vi "ActiView806-Lores.vi"() -> ()   [LabVIEW 2020] (continued)
          tunnel: [i32[] [1, 2, 3] ("Disabled Items []") i32[] [2, 3] ("Disabled Items []") i32[] [3] ("Disabled Items []") i32[] [] ("Disabled Items []") i32[] [1, 2, 3] ("Disabled Items []") i32[] [2, 3] ("Disabled Items []")] -> w1444
          tunnel: [u32 1 u32 3 u32 7 u32 15 u32 1 u32 3] -> w1438
          frame 0, Default {
          }
          frame 1 {
          }
          frame 2 {
          }
          frame 3 {
          }
          frame 14 {
          }
          frame 15 {
          }
        }
        n877 = local read "MonFreeAvg2"() -> (w1602:i32)
        n878 = local read "RefFreeAvg2"() -> (w1607:i32[])
        n879 = local read "MonFreeAvg1"() -> (w1597:i32)
        n880 = for {
          tunnel: w1584 -> [w2146]
          shift-right: [w2142] -> w1592
          shift-left: i32[] [] -> [w2144]
          tunnel: w1608 -> [w2140] mode=indexing
          n881 = Search 1D Array(1D array=w2146, element=w2140) -> (index of element=w2145:i32)  [unwired: 1 out]
          n882 = Greater Or Equal To 0?(x=w2145) -> (x >= 0?=w2143:bool)
          n883 = Build Array (concatenate)(w2144, w2140) -> (w2141:i32[])
          n884 = Select(t=w2141, s=w2143, f=w2144) -> (s? t:f=w2142:i32[])
        }
        n885 = for {
          tunnel: w1584 -> [w2139]
          shift-right: [w2135] -> w1586
          shift-left: i32[] [] -> [w2137]
          tunnel: w1607 -> [w2133] mode=indexing
          n886 = Search 1D Array(1D array=w2139, element=w2133) -> (index of element=w2138:i32)  [unwired: 1 out]
          n887 = Greater Or Equal To 0?(x=w2138) -> (x >= 0?=w2136:bool)
          n888 = Build Array (concatenate)(w2137, w2133) -> (w2134:i32[])
          n889 = Select(t=w2134, s=w2136, f=w2137) -> (s? t:f=w2135:i32[])
        }
        n890 = Search 1D Array(1D array=w1584, element=w1602) -> (index of element=w1604:i32)  [unwired: 1 out]
        n891 = Search 1D Array(1D array=w1584, element=w1597) -> (index of element=w1600:i32)  [unwired: 1 out]
        n892 = Greater Or Equal To 0?(x=w1604) -> (x >= 0?=w1603:bool)
        n893 = Greater Or Equal To 0?(x=w1600) -> (x >= 0?=w1599:bool)
        n894 = Select(t=w1438, s=w1439, f=u32 1) -> (s? t:f=w1440:u32)
        n895 = Select(t=w1602, s=w1603, f=0) -> (s? t:f=w1595:i32)
        n896 = Select(t=w1597, s=w1599, f=0) -> (s? t:f=w1596:i32)
        n897 = property on="Box" class="Ring (strict)"("Visible"=w1439, "Disabled Items []"=w1444) -> ()  [unwired: 2 in, 2 out]
        n898 = Bundle By Name(cluster=w1442, "Save Box"=w1440) -> (w1441:T7)
        n899 = Array Size(array=w1592) -> (size(s)=w1594:i32)
        n900 = Array Size(array=w1586) -> (size(s)=w1589:i32)
        n901 = Equal To 0?(x=w1594) -> (x = 0?=w1593:bool)
        n902 = Equal To 0?(x=w1589) -> (x = 0?=w1588:bool)
        n903 = Select(t=i32[] [0], s=w1593, f=w1592) -> (s? t:f=w1591:i32[])
        n904 = Select(t=i32[] [0], s=w1588, f=w1586) -> (s? t:f=w1585:i32[])
        n905 = case shown="True" w1625 {
          tunnel: w1647 -> [_ w2249]
          tunnel: w1579 -> [_ w2248]
          tunnel: w1578 -> [_ w2247]
          tunnel: w1613 -> [_ w2246]
          tunnel: w1639 -> [_ w2245]
          tunnel: w1577 -> [_ w2244]
          tunnel: w1643 -> [_ w2243]
          tunnel: w1636 -> [_ w2242]
          tunnel: w1596 -> [_ w2241]
          tunnel: w1591 -> [_ w2240]
          tunnel: w1595 -> [_ w2239]
          tunnel: w1585 -> [_ w2238]
          tunnel: w1574 -> [_ w2235]
          tunnel: w1573 -> [_ w2237]
          tunnel: w1439 -> [_ w2233]
          tunnel: w1474 -> [_ w2231]
          frame False {
          }
          frame True {
            w2236 = i8 7 items=["A1 - H32 (256)", "A1 - E32 (160)", "A1 - D32 (128)", "A1 - B32 (64)", "A1 - A32 (32)", "A1 - A16 (16)", "A1 -A8 (8)", "None (0) "] ("TCPsubset")
            n906 = local write "Channels"(w2249) -> ()
            n907 = local write "Offset"(w2245) -> ()
            n908 = local write "Reference"(w2243) -> ()
            n909 = property on="Channels" class="Ring (strict)"("Disabled Items []"=w2248) -> ()  [unwired: 2 in, 2 out]
            n910 = property on="Reference" class="Ring (strict)"("Disabled Items []"=w2247) -> ()  [unwired: 2 in, 2 out]
            n911 = property on="Offset" class="Ring (strict)"("Disabled Items []"=w2244) -> ()  [unwired: 2 in, 2 out]
            n912 = property on="TCPsubset" class="Ring (strict)"("Disabled Items []"=w2237) -> ()  [unwired: 2 in, 2 out]
            n913 = local write "MonFree"(w2246) -> ()
            n914 = Select(t=w2236, s=w2233, f=w2235) -> (s? t:f=w2234:i8)
            n915 = local write "RefFree"(w2242) -> ()
            n916 = local write "TCPsubset"(w2234) -> ()
            n917 = local write "MonFreeAvg1"(w2241) -> ()
            n918 = local read "AddTP"() -> (w2229:bool)
            n919 = local write "RefFreeAvg1"(w2240) -> ()
            n920 = local write "Charts/Graphs"(T2."Monopolar Display" ("Charts/Graphs")) -> ()
            n921 = local write "MonFreeAvg2"(w2239) -> ()
            n922 = And(x=w2229, y=w2231) -> (x .and. y?=w2230:bool)
            n923 = local write "AddTP"(w2230) -> ()
            n924 = local write "RefFreeAvg2"(w2238) -> ()
          }
        }
        n925 = local read "TCPaddTP"() -> (w1534:bool)
        n926 = local read "TCPaddAnas"() -> (w1530:bool)
        n927 = local read "TCPaddTrig"() -> (w1526:bool)
        n928 = local read "TCPaddSens"() -> (w1532:bool)
        n929 = local read "TCPaddJazz"() -> (w1473:bool)
        n930 = local read "Averaging"() -> (w1528:bool)
        n931 = Not(x=w1439) -> (.not. x?=w1472:bool)
        n932 = And(x=w1472, y=w1528) -> (x .and. y?=w1527:bool)
        n933 = Compound Arithmetic op=AND(w1534, w1474, w1472) -> (w1533:bool)
        n934 = Compound Arithmetic op=AND(w1532, w1474, w1472) -> (w1531:bool)
        n935 = Compound Arithmetic op=AND(w1530, w1496, w1472) -> (w1529:bool)
        n936 = And(x=w1526, y=w1472) -> (x .and. y?=w1525:bool)
        n937 = Compound Arithmetic op=AND(w1473, w1470, w1472) -> (w1471:bool)
        n938 = local write "Averaging"(w1527) -> ()
        n939 = local write "TCPaddTP"(w1533) -> ()
        n940 = local write "TCPaddAnas"(w1529) -> ()
        n941 = local write "TCPaddTrig"(w1525) -> ()
        n942 = local write "TCPaddSens"(w1531) -> ()
        n943 = local write "TCPaddJazz"(w1471) -> ()
        n944 = property on="Charts/Graphs" class="TabCtl (strict)"() -> ("Pages"=w1557:refnum<vi>[])  [unwired: 2 in, 2 out]
        n945 = Index Array(array=w1557, index #1=1 ("index")) -> (element #1=w1550:refnum<vi>, element #3=w1536:refnum<vi>, element #4=w1549:refnum<vi>, element #5=w1491:refnum<vi>, element #6=w1492:refnum<vi>, element #7=w1535:refnum<vi>)  [unwired: 6 in, 1 out]
        n946 = Array Size(array=w1569) -> (size(s)=w1635:i32)
        n947 = Unbundle By Name(w1633) -> ("All Labels"=w1486:string[])
        n948 = Not Equal To 0?(x=w1635) -> (x != 0?=w1634:bool)
        n949 = Unbundle By Name(w1441) -> ("Mon Channels"=w1658:i32, "Bip Channels"=w1657:i32, "Aux Channels"=w1567:i32, "Jazz Channels"=w1485:i32, "Ana Channels"=w1490:i32)
        n950 = And(x=w1634, y=w1474) -> (x .and. y?=w1541:bool)
        n951 = Array Size(array=w1542) -> (size(s)=w1559:i32)
        n952 = Array Size(array=w1480) -> (size(s)=w1481:i32)
        n953 = Array Size(array=w1543) -> (size(s)=w1561:i32)
        n954 = property on="Ring Buffer" class="Knob (strict)"("Scale.Uniform Marker Spacing?"=FALSE) -> ()  [unwired: 2 in, 2 out]
        n955 = Not Equal To 0?(x=w1481) -> (x != 0?=w1478:bool)
        n956 = Not Equal To 0?(x=w1559) -> (x != 0?=w1558:bool)
        n957 = Not Equal To 0?(x=w1561) -> (x != 0?=w1560:bool)
        n958 = Array Size(array=w1486) -> (size(s)=w1632:i32)
        n959 = Select(t=T5."Enabled" ("Disabled"), s=w1541, f=T5."Disabled and Grayed Out" ("Disabled")) -> (s? t:f=w1568:T5)
        n960 = And(x=w1560, y=w1496) -> (x .and. y?=w1545:bool)
        n961 = And(x=w1478, y=w1470) -> (x .and. y?=w1479:bool)
        n962 = And(x=w1558, y=w1474) -> (x .and. y?=w1551:bool)
        n963 = Select(t=T4."Page Enabled" ("Page Enabled State"), s=w1541, f=T4."Page Disabled & Grayed" ("Page Enabled State")) -> (s? t:f=w1555:T4)
        n964 = Select(t=T4."Page Enabled" ("Page Enabled State"), s=w1479, f=T4."Page Disabled & Grayed" ("Page Enabled State")) -> (s? t:f=w1497:T4)
        n965 = Decrement(x=w1632) -> (x-1=w1631:i32)
        n966 = Select(t=T4."Page Enabled" ("Page Enabled State"), s=w1545, f=T4."Page Disabled & Grayed" ("Page Enabled State")) -> (s? t:f=w1546:T4)
        n967 = Select(t=T4."Page Enabled" ("Page Enabled State"), s=w1551, f=T4."Page Disabled & Grayed" ("Page Enabled State")) -> (s? t:f=w1548:T4)
        n968 = Select(t=T4."Page Enabled" ("Page Enabled State"), s=w1472, f=T4."Page Disabled & Grayed" ("Page Enabled State")) -> (s? t:f=w1537:T4)
        n969 = property on="TP Offset Graph 1" class="WFGraph (strict)"("Disabled"=w1568) -> ()  [unwired: 2 in, 2 out]
        n970 = property on="TP Offset Graph 2" class="WFGraph (strict)"("Disabled"=w1568) -> ()  [unwired: 2 in, 2 out]
        n971 = Index Array(array=w1486, index=w1631) -> (element=w1489:string)
        n972 = property class="Page"(reference=w1550, "Page Enabled State"=w1555) -> ()  [unwired: 1 in, 2 out]
        n973 = property class="Page"(reference=w1549, "Page Enabled State"=w1548) -> ()  [unwired: 1 in, 2 out]
        n974 = property class="Page"(reference=w1491, "Page Enabled State"=w1497) -> ()  [unwired: 1 in, 2 out]
        n975 = property class="Page"(reference=w1492, "Page Enabled State"=w1546) -> ()  [unwired: 1 in, 2 out]
        n976 = property class="Page"(reference=w1536, "Page Enabled State"=w1537) -> ()  [unwired: 1 in, 2 out]
        n977 = property class="Page"(reference=w1535, "Page Enabled State"=w1537) -> ()  [unwired: 1 in, 2 out]
        n978 = Array Subset(array=w1486, length=w1658) -> (w1663:string[])  [unwired: 1 in]
        n979 = Array Subset(array=w1486, index=256, length=w1657) -> (w1662:string[])
        n980 = Array Subset(array=w1486, index=264, length=w1567) -> (w1659:string[])
        n981 = Array Subset(array=w1486, index=272, length=w1485) -> (w1487:string[])
        n982 = Array Subset(array=w1486, index=281, length=w1490) -> (w1488:string[])
        n983 = Build Array (concatenate)(w1663, w1662, w1659, w1487, w1488, w1489) -> (w1630:string[])
        n984 = for {
          N: w1464 -> [_]
          tunnel: w1630 -> [w2251] mode=indexing
          tunnel: [w2250] -> w1672 mode=indexing
          n985 = String Subset(string=w2251, length (rest)=4 ("length (rest)")) -> (substring=w2250:string)  [unwired: 1 out]
        }
        n986 = for {
          tunnel: w1630 -> [w2219] mode=indexing
          tunnel: [w2218] -> w1628 mode=indexing
          n987 = Format Into String(format string="%-16.16s", w2219) -> (resulting string=w2218:string)  [unwired: 2 in, 1 out]
        }
        n988 = property on="MonFree" class="LstBox (strict)"("Item Names"=w1672) -> ()  [unwired: 2 in, 2 out]
        n989 = property on="RefFree" class="LstBox (strict)"("Item Names"=w1672) -> ()  [unwired: 2 in, 2 out]
        n990 = Bundle By Name(cluster=w1633, "Spec Labels"=w1628) -> (w1629:T8)
        n991 = Select(t=T5."Enabled" ("Disabled"), s=w1474, f=T5."Disabled and Grayed Out" ("Disabled")) -> (s? t:f=w1671:T5)
        n992 = property on="RefFreeAvg1" class="LstBox (strict)"("Item Names"=w1672) -> ()  [unwired: 2 in, 2 out]
        n993 = property on="MonFreeAvg1" class="LstBox (strict)"("Item Names"=w1672) -> ()  [unwired: 2 in, 2 out]
        n994 = property on="Battery\nCapacitance" class="Slide (strict)"("Disabled"=w1671) -> ()  [unwired: 2 in, 2 out]
        n995 = property on="RefFreeAvg2" class="LstBox (strict)"("Item Names"=w1672) -> ()  [unwired: 2 in, 2 out]
        n996 = property on="MonFreeAvg2" class="LstBox (strict)"("Item Names"=w1672) -> ()  [unwired: 2 in, 2 out]
      }
      frame 2 {
        w2260 = T5."Disabled and Grayed Out" ("Disabled")
        w2294 = 5  # Go to State 5:    stop running
        w2266 = FALSE
        w2261 = FALSE
        w2278 = 0 ("Dimension Size")
        w2307 = FALSE  # Stop Running
        w2310 = 4  # Go to State 4    Displaying
        w2311 = 3  # Go to State 3     Saving
        # "Screen Duration"
        # "Sample Rate"
        # "Busy Saving"
        n997 = flat-sequence {
          tunnel: w2273 -> [w2318]
          tunnel: w2271 -> [w2317]
          tunnel: w2272 -> [w2316]
          tunnel: w2271 -> [w2323]
          tunnel: w2271 -> [w2328]
          frame #0 {
            w2314 = 0 ("Dimension Size")
            # "Cear the Charts"
            n998 = Initialize Array(w2314, w2314, w2314) -> (w2313:i32[][])
            n999 = To Double Precision Float(number=w2313) -> (double precision float=w2312:dbl[][])
            n1000 = property on="Trigger Chart" class="WFChart (strict)"("History Data"=w2313) -> ()  [unwired: 2 in, 2 out]
            n1001 = property on="Mon Chart" class="WFChart (strict)"("History Data"=w2312) -> ()  [unwired: 2 in, 2 out]
            n1002 = property on="Bip Chart" class="WFChart (strict)"("History Data"=w2312) -> ()  [unwired: 2 in, 2 out]
            n1003 = property on="Aux Chart" class="WFChart (strict)"("History Data"=w2312) -> ()  [unwired: 2 in, 2 out]
            n1004 = property on="Jazz Chart" class="WFChart (strict)"("History Data"=w2312) -> ()  [unwired: 2 in, 2 out]
            n1005 = property on="Ana Chart" class="WFChart (strict)"("History Data"=w2312) -> ()  [unwired: 2 in, 2 out]
          }
          frame #1 {
            # "Scale the Charts"
            # "Set \"Chart History Lenght\" at:\n(x-scale lenghts in s) * (sample rate) + 1"
            # "Sample Rate on screen"
            n1006 = Multiply(x=w2316, y=w2317) -> (x*y=w2321:i32)
            n1007 = Quotient & Remainder(x=w2318, y=w2321) -> (floor(x/y)=w2320:i32)  [unwired: 1 out]
            n1008 = To Double Precision Float(number=w2320) -> (double precision float=w2319:dbl)
            n1009 = Reciprocal(x=w2319) -> (1/x=w2315:dbl)
            n1010 = property on="Mon Chart" class="WFChart (strict)"("X Scale.Offset and Multiplier:Multiplier"=w2315) -> ()  [unwired: 2 in, 2 out]
            n1011 = property on="Trigger Chart" class="WFChart (strict)"("X Scale.Offset and Multiplier:Multiplier"=w2315) -> ()  [unwired: 2 in, 2 out]
            n1012 = property on="Bip Chart" class="WFChart (strict)"("X Scale.Offset and Multiplier:Multiplier"=w2315) -> ()  [unwired: 2 in, 2 out]
            n1013 = property on="Aux Chart" class="WFChart (strict)"("X Scale.Offset and Multiplier:Multiplier"=w2315) -> ()  [unwired: 2 in, 2 out]
            n1014 = property on="Jazz Chart" class="WFChart (strict)"("X Scale.Offset and Multiplier:Multiplier"=w2315) -> ()  [unwired: 2 in, 2 out]
            n1015 = property on="Ana Chart" class="WFChart (strict)"("X Scale.Offset and Multiplier:Multiplier"=w2315) -> ()  [unwired: 2 in, 2 out]
          }
          frame #2 {
            n1016 = To Double Precision Float(number=w2323) -> (double precision float=w2322:dbl)
            n1017 = property on="Mon Chart" class="WFChart (strict)"("X Scale.Range:Maximum"=w2322) -> ()  [unwired: 2 in, 2 out]
            n1018 = property on="Trigger Chart" class="WFChart (strict)"("X Scale.Range:Maximum"=w2322) -> ()  [unwired: 2 in, 2 out]
            n1019 = property on="Bip Chart" class="WFChart (strict)"("X Scale.Range:Maximum"=w2322) -> ()  [unwired: 2 in, 2 out]
            n1020 = property on="Aux Chart" class="WFChart (strict)"("X Scale.Range:Maximum"=w2322) -> ()  [unwired: 2 in, 2 out]
            n1021 = property on="Jazz Chart" class="WFChart (strict)"("X Scale.Range:Maximum"=w2322) -> ()  [unwired: 2 in, 2 out]
            n1022 = property on="Ana Chart" class="WFChart (strict)"("X Scale.Range:Maximum"=w2322) -> ()  [unwired: 2 in, 2 out]
          }
          frame #3 {
            n1023 = Greater Or Equal?(x=1, y=w2328) -> (x >= y?=w2327:bool)
            n1024 = Select(t=u8 1, s=w2327, f=u8 0) -> (s? t:f=w2324:u8)
            n1025 = property on="Mon Chart" class="WFChart (strict)"("X Scale.Format & Precision:Precision"=w2324) -> ()  [unwired: 2 in, 2 out]
            n1026 = property on="Bip Chart" class="WFChart (strict)"("X Scale.Format & Precision:Precision"=w2324) -> ()  [unwired: 2 in, 2 out]
            n1027 = property on="Aux Chart" class="WFChart (strict)"("X Scale.Format & Precision:Precision"=w2324) -> ()  [unwired: 2 in, 2 out]
            n1028 = property on="Jazz Chart" class="WFChart (strict)"("X Scale.Format & Precision:Precision"=w2324) -> ()  [unwired: 2 in, 2 out]
            n1029 = property on="Ana Chart" class="WFChart (strict)"("X Scale.Format & Precision:Precision"=w2324) -> ()  [unwired: 2 in, 2 out]
          }
        }
        n1030 = Unbundle By Name(w2267) -> ("ADC Rate"=w2273:i32, "Screen Ratio"=w2272:i32)
        n1031 = for {
          N: 9 -> [_]
          tunnel: w2300 -> [w2353]
          tunnel: [w2349] -> w2301 mode=indexing
          i -> [w2354]
          n1032 = Multiply(x=w2353, y=w2354) -> (x*y=w2352:i32)
          n1033 = To Double Precision Float(number=w2352) -> (double precision float=w2351:dbl)
          n1034 = Bundle(w2351, u32 0) -> (w2349:cluster{dbl, u32})  [unwired: 1 out]
        }
        n1035 = property on="Ring Buffer" class="Knob (strict)"("Scale.Marker Values[]"=w2301) -> ()  [unwired: 2 in, 2 out]
        n1036 = property on="ScreenLength" class="Ring (strict)"("Disabled"=w2260) -> ()  [unwired: 2 in, 2 out]
        n1037 = property on="Decimation" class="Ring (strict)"("Disabled"=w2260) -> ()  [unwired: 2 in, 2 out]
        n1038 = property on="Buffer" class="Ring (strict)"("Disabled"=w2260) -> ()  [unwired: 2 in, 2 out]
        n1039 = property on="Load Configuration File" class="Bool"("Disabled"=w2260) -> ()  [unwired: 2 in, 2 out]
        n1040 = property on="Save Configuration File" class="Bool"("Disabled"=w2260) -> ()  [unwired: 2 in, 2 out]
        n1041 = property on="Edit" class="Bool"("Disabled"=w2260) -> ()  [unwired: 2 in, 2 out]
        n1042 = property on="LocalPort" class="DigNum (strict)"("Disabled"=w2260) -> ()  [unwired: 2 in, 2 out]
        n1043 = property on="TCPsubset" class="Ring (strict)"("Disabled"=w2260) -> ()  [unwired: 2 in, 2 out]
        n1044 = property on="TCPaddTP" class="Bool (strict)"("Disabled"=w2260) -> ()  [unwired: 2 in, 2 out]
        n1045 = property on="TCPaddSens" class="Bool (strict)"("Disabled"=w2260) -> ()  [unwired: 2 in, 2 out]
        n1046 = property on="TCPaddAnas" class="Bool (strict)"("Disabled"=w2260) -> ()  [unwired: 2 in, 2 out]
        n1047 = property on="TCPaddJazz" class="Bool (strict)"("Disabled"=w2260) -> ()  [unwired: 2 in, 2 out]
        n1048 = property on="TCPaddTrig" class="Bool (strict)"("Disabled"=w2260) -> ()  [unwired: 2 in, 2 out]
        n1049 = property on="JazzOn" class="Bool (strict)"("Disabled"=w2260) -> ()  [unwired: 2 in, 2 out]
        n1050 = global write "TCPidentification.glb" "TCP cluster"(T9 {"connection ID"=refnum, "remote address"="", "remote port"=0} ("TCP cluster")) -> ()
        n1051 = local write "Save Subset"("" ("Local Patient Identification")) -> ()
        n1052 = local write "with  8 EX"(w2266) -> ()
        n1053 = local write "with Sens"(w2266) -> ()
        n1054 = local write "with AIB"(w2266) -> ()
        n1055 = local write "RejAbs"(w2266) -> ()
        n1056 = local write "RejDif"(w2266) -> ()
        n1057 = local write "Box1"(w2266) -> ()
        n1058 = local write "Box2"(w2266) -> ()
        n1059 = local write "Box3"(w2266) -> ()
        n1060 = local write "Box4"(w2266) -> ()
        n1061 = Greater Than 0?(x=w2277) -> (x > 0?=w2276:bool)
        n1062 = Unbundle By Name(w2267) -> ("Mon Channels"=w2292:i32, "Bip Channels"=w2291:i32)
        n1063 = property on="MonFree" class="LstBox (strict)"() -> ("Item Names"=w2282:string[])  [unwired: 2 in, 2 out]
        n1064 = To Double Precision Float(number=w2278) -> (double precision float=w2281:dbl)
        n1065 = local write "Total Saved sec"(w2278) -> ()
        n1066 = case shown="True" w2276 {
          tunnel: w2277 -> [_ w2342]
          frame False {
          }
          frame True {
            n1067 = Divide(x=w2342, y=2.0) -> (x/y=w2344:dbl)
            n1068 = Decrement(x=w2344) -> (x-1=w2332:dbl)
            n1069 = property on="BipLPfreq" class="DigNum (strict)"("Data Range:Maximum"=w2332) -> ()  [unwired: 2 in, 2 out]
            n1070 = property on="AvgLPfreq" class="DigNum (strict)"("Data Range:Maximum"=w2332) -> ()  [unwired: 2 in, 2 out]
            n1071 = property on="MonLPfreq" class="DigNum (strict)"("Data Range:Maximum"=w2332) -> ()  [unwired: 2 in, 2 out]
            n1072 = property on="AnaHPfreq" class="DigNum (strict)"("Data Range:Maximum"=w2332) -> ()  [unwired: 2 in, 2 out]
            n1073 = local read "MonLPfreq"() -> (w2341:dbl)
            n1074 = local read "AvgLPfreq"() -> (w2335:dbl)
            n1075 = local read "AnaLPfreq"() -> (w2331:dbl)
            n1076 = local read "BipLPfreq"() -> (w2338:dbl)
            n1077 = Less Or Equal?(x=w2338, y=w2332) -> (x <= y?=w2339:bool)
            n1078 = Less Or Equal?(x=w2341, y=w2332) -> (x <= y?=w2345:bool)
            n1079 = Less Or Equal?(x=w2335, y=w2332) -> (x <= y?=w2336:bool)
            n1080 = Less Or Equal?(x=w2331, y=w2332) -> (x <= y?=w2333:bool)
            n1081 = Select(t=w2338, s=w2339, f=w2332) -> (s? t:f=w2337:dbl)
            n1082 = Select(t=w2341, s=w2345, f=w2332) -> (s? t:f=w2340:dbl)
            n1083 = Select(t=w2335, s=w2336, f=w2332) -> (s? t:f=w2334:dbl)
            n1084 = Select(t=w2331, s=w2333, f=w2332) -> (s? t:f=w2330:dbl)
            n1085 = local write "MonLPfreq"(w2340) -> ()
            n1086 = local write "BipLPfreq"(w2337) -> ()
            n1087 = local write "AnaLPfreq"(w2330) -> ()
            n1088 = local write "AvgLPfreq"(w2334) -> ()
          }
        }
        n1089 = global write "LoBatWarning.glb" "LoBatWarning"(w2261) -> ()
        n1090 = global write "JazzLoBatWarning.glb" "JazzLoBatWarning"(w2261) -> ()
        n1091 = Format Into String(format string="%-4.4s", "" ("input 1")) -> (resulting string=w2284:string)  [unwired: 2 in, 1 out]
        n1092 = global write "StopThreads.glb" "StopThreads"(w2261) -> ()
        n1093 = property class="VI"("Front Panel Window:Closeable"=FALSE) -> ()  [unwired: 2 in, 2 out]
        n1094 = local write "Current File MB"(w2281) -> ()
        n1095 = Build Array (concatenate)(w2282, w2284) -> (w2288:string[])
        n1096 = Add(x=w2292, y=w2291) -> (x+y=w2290:i32)
        n1097 = Match First String(2:w2288, 3:w2284) -> (0:w2289:i32)  [unwired: 1 out]
        n1098 = Not Equal?(x=w2289, y=w2290) -> (x != y?=w2283:bool)
        n1099 = Build Array(FALSE ("element"), w2283, FALSE ("element")) -> (w2303:bool[])
        n1100 = case shown="True" w2262 {
          selector: w2262 -> [_ w2346]
          frame False {
          }
          frame True {
            n1101 = flat-sequence {
              tunnel: w2346 -> [w2347]
              frame #0 {
                n1102 = local write "Start Saving"(w2347) -> ()
              }
              frame #1 {
                n1103 = property on="Start Saving" class="Bool (strict)"("Boolean Text.Text"="Initializing") -> ()  [unwired: 2 in, 2 out]
              }
            }
          }
        }
        n1104 = Boolean Array To Number(Boolean array=w2303) -> (number=w2298:u32)
        n1105 = call "Act_ConfigError.vi"("Error Code In"=w2298, "error in (no error)"=w2297) -> ("error out"=w2264:errorcluster)  [unwired: 2 out]
        n1106 = Unbundle By Name(w2264) -> ("status"=w2296:bool)
        n1107 = Select(t=w2311, s=w2262, f=w2310) -> (s? t:f=w2295:i32)
        n1108 = Select(t=w2294, s=w2296, f=w2295) -> (s? t:f=w2293:i32)
      }
      frame 3 {
        w2411 = 43 items=["No Error", "Manager Argument Error", "Memory Full", "Out of Zone", "End of File", "File Already Open", "Generic File IO Error", "File Not Found", "File Permission Error", "Disk Full", "Duplicate Path", "Too Many Files Open", "Not Enabled", "Resource File Not Found", "Cannot Add Resource", "Resource Not Found", "Image Not Found", "Image Memory Error", "Pen Does Not Exist", "Config Bad Type", "Config Token Not Found", "Config Parse Error", "Config Memory Error", "Bad External Code Format", "Bad External Code Offset", "External Code Not Present", "Null Window", "Destroy Window Mixup", "Null Menu", "Print Aborted", "Bad Print Record", "Print Driver Error", "Windows Error During Print", "Memory Error During Print", "Print Dialog Error", "Generic Print Error", "Invalid Device Refnum", "Device Not Found", "Device Parameter Error", "Device Unit Error", "Can't Open Device", "Device Call Aborted", "Generic Error", "Cancelled By User"]
        w2426 = 43 items=["No Error", "Manager Argument Error", "Memory Full", "Out of Zone", "End of File", "File Already Open", "Generic File IO Error", "File Not Found", "File Permission Error", "Disk Full", "Duplicate Path", "Too Many Files Open", "Not Enabled", "Resource File Not Found", "Cannot Add Resource", "Resource Not Found", "Image Not Found", "Image Memory Error", "Pen Does Not Exist", "Config Bad Type", "Config Token Not Found", "Config Parse Error", "Config Memory Error", "Bad External Code Format", "Bad External Code Offset", "External Code Not Present", "Null Window", "Destroy Window Mixup", "Null Menu", "Print Aborted", "Bad Print Record", "Print Driver Error", "Windows Error During Print", "Memory Error During Print", "Print Dialog Error", "Generic Print Error", "Invalid Device Refnum", "Device Not Found", "Device Parameter Error", "Device Unit Error", "Can't Open Device", "Device Call Aborted", "Generic Error", "Cancelled By User"]
        w2441 = FALSE  # Stop Running
        # "Jazz Chan Selection"
        # "Ana Chan Selection"
        # "Aux Chan Selection"
        # "Mon Chan Selection"
        # "path does exist"
        # "Current File in Byte"
        # "Header Lenght in Byte"
        n1109 = Unbundle By Name(w2414) -> ("Save Path"=w2362:path, "Mark2"=w2374:bool, "GSR16Hz"=w2373:bool, "Jazz Channels"=w2372:i32, "Speed Mode"=w2364:i8, "ADC Rate"=w2418:i32, "Decimate Ratio"=w2419:i32, "Mon Channels"=w2400:i32, "Bip Channels"=w2399:i32, "Save Subset"=w2398:i8, "Add Touchproofs"=w2397:bool, "Add Sensors"=w2393:bool, "Add Jazz"=w2379:bool, "Add Anas"=w2380:bool, "Save Box"=w2381:u32)
        n1110 = Not Equal To 0?(x=w2372) -> (x != 0?=w2367:bool)
        n1111 = call "AVTCP-Local ID FGV.vi"() -> ("Value out"=w2357:cluster{"subj":string, "rec":string}, "not empty"=w2358:bool)  [unwired: 6 in]
        n1112 = Bundle("Save Subset"=w2398, "Add Touchproofs"=w2397, "Add Sensors"=w2393, "Add Jazz"=w2379, "Add Anas"=w2380, "Save Box"=w2381) -> (w2424:T20)  [unwired: 1 out]
        n1113 = case shown="False" w2358 {
          tunnel: [w2453 w2455] -> w2437
          tunnel: w2424 -> [w2452 w2456]
          tunnel: [w2451 w2456] -> w2413
          tunnel: [w2450 "Default" ("Save Subset")] -> w2406
          tunnel: w2374 -> [w2449 _]
          tunnel: [w2448 _] -> w2368
          tunnel: w2367 -> [w2447 _]
          tunnel: w2364 -> [w2446 _]
          tunnel: w2357 -> [_ w2455]
          frame False {
            n1114 = call "BDFlocal-Daisy.vi"("Mark2"=w2449, "JazzOn"=w2447, "Speedmode"=w2446, "Default Save Cluster"=w2452) -> ("Save Subset"=w2450:string, "Local ID"=w2453:T21, "Save Cluster"=w2451:T20, "error out"=w2448:errorcluster)
          }
          frame True {
          }
        }
        n1115 = Bundle("Mark2"=w2374, "GSR16Hz"=w2373, w2367, "Speed Mode"=w2364) -> (w2405:T22)  [unwired: 1 out]
        n1116 = Strip Path(path=w2362) -> (stripped path=w2370:path, name=w2385:string)
        n1117 = Unbundle By Name(w2368) -> ("code"=w2412:i32)
        n1118 = File/Directory Info(path=w2370, error in=w2368) -> (directory=w2369:bool)  [unwired: 6 out]
        n1119 = call "AVTCP-Filepath FGV.vi"() -> ("Value out"=w2359:path)  [unwired: 7 in]
        n1120 = call "AVTCP-TCP Options FGV.vi"() -> ("Value out"=w2355:T23, "not empty"=w2356:bool)  [unwired: 6 in]
        n1121 = Empty String/Path?(string/path=w2359) -> (empty?=w2361:bool)
        n1122 = case shown="True" w2356 {
          tunnel: w2355 -> [_ w2445]
          frame False {
          }
          frame True {
            n1123 = Unbundle By Name(w2445) -> ("Subset"=w2444:i32, "EX"=w2443:bool)
            n1124 = local write "TCPsubset"(w2444) -> ()
            n1125 = local write "TCPaddTP"(w2443) -> ()
            n1126 = local write "TCPaddTrig"(TRUE ("TCPaddTrig")) -> ()
          }
        }
        n1127 = Equal?(x=w2412, y=w2411) -> (x = y?=w2409:bool)
        n1128 = Not(x=w2361) -> (.not. x?=w2360:bool)
        n1129 = Unbundle By Name(w2413) -> ("Save Subset"=w2403:i8, "Add Touchproofs"=w2401:bool, "Add Sensors"=w2396:bool, "Add Jazz"=w2376:bool, "Add Anas"=w2377:bool, "Save Box"=w2378:u32)
        n1130 = Compound Arithmetic op=OR(w2360, w2369, w2409) -> (w2410:bool)
        n1131 = case shown="False" w2410 {
          tunnel: [w2467 w2479] -> w2388
          tunnel: w2368 -> [w2469 w2478]
          tunnel: w2370 -> [_ w2479]
          tunnel: [w2474 w2478] -> w2386
          frame False {
            w2467 = path ""  # Empty Path
            w2477 = T18 1 items=["no dialog", "OK message", "continue or stop message", "OK message + warnings", "continue/stop + warnings"] ("type of dialog (OK msg:1)")
            w2474 = errorcluster {"status"=FALSE, "code"=0, "source"=""}  # No Error
            w2472 = FALSE ("element")
            n1132 = Build Array(w2472, w2472, w2472, TRUE ("element")) -> (w2473:bool[])
            n1133 = Boolean Array To Number(Boolean array=w2473) -> (number=w2470:u32)
            n1134 = call "Act_ConfigError.vi"("Error Code In"=w2470, "error in (no error)"=w2469) -> ("[user-defined descriptions]"=w2475:string[], "[user-defined codes]"=w2476:i32[], "error out"=w2468:errorcluster)
            n1135 = call <vilib>:"General Error Handler.vi"("[user-defined codes]"=w2476, "[user-defined descriptions]"=w2475, "type of dialog (OK msg:1)"=w2477, "error in (no error)"=w2468) -> ()  [unwired: 1 in, 11 out]
          }
          frame True {
          }
        }
        n1136 = Empty String/Path?(string/path=w2359) -> (empty?=w2363:bool)
        n1137 = case shown="True" w2363 {
          tunnel: [w2458 w2466] -> w2389
          tunnel: w2388 -> [_ w2465]
          tunnel: [w2457 w2464] -> w2387
          tunnel: w2386 -> [w2457 w2463]
          tunnel: w2385 -> [_ w2462]
          tunnel: w2359 -> [w2458 _]
          frame False {
          }
          frame True {
            n1138 = File Dialog(4:"BioSemi Data Format" ("pattern label"), 6:"*.bdf" ("pattern (all files)"), 7:"Enter filename:" ("prompt"), 8:w2463, 9:w2462, 11:w2465) -> (0:w2464:errorcluster, 3:w2466:path)  [unwired: 3 out]
          }
        }
        n1139 = Unbundle By Name(w2417) -> ("ElecGain"=w2371:i8, "BreathBelt"=w2366:i8)
        n1140 = Bundle("Speed Mode"=w2364, "Save Subset"=w2403, "Initially Channel Selection"=w2402, "Add Touchproofs"=w2401, "Mon Channels"=w2400, "Bip Channels"=w2399, "Add Sensors"=w2396, "Initially Channel Selection"=w2395, "Add Jazz"=w2376, "Initially Channel Selection"=w2375, "Add Anas"=w2377, "Initially Channel Selection"=w2394, "Save Box"=w2378) -> (w2365:T17)  [unwired: 1 out]
        n1141 = Open/Create/Replace File(file path (use dialog)=w2389, error in=w2387, operation (0:open)=T10."replace or create with confirmation") -> (refnum out=w2391:refnum<file>, error out=w2390:errorcluster)  [unwired: 4 out]
        n1142 = Initialize Array(u8 255, 1) -> (w2433:u8[])
        n1143 = call "Write File+ [U8].vi"("1D array"=w2433, "error in (no error)"=w2390, "refnum"=w2391) -> ("error out"=w2438:errorcluster, "dup refnum"=w2439:refnum<file>)  [unwired: 2 in, 2 out]
        n1144 = Unbundle By Name(w2440) -> ("Spec Labels"=w2436:string[])
        n1145 = Array Size(array=w2433) -> (size(s)=w2423:i32)
        n1146 = call "SaveSelectDaisy.vi"("Save Selection Cluster"=w2365) -> ("ChanSelection"=w2404:i32[])  [unwired: 1 out]
        n1147 = call "BDFheader.vi"("ElecGain"=w2371, "BreathBelt"=w2366, "ChanSelection"=w2404, "Configuration"=w2405, "BDF Label Array"=w2436, "Decimate Ratio"=w2419, "ADC Sample Rate"=w2418, "Local ID"=w2437, "PreHeader Lenght"=w2423) -> ("BDF header Out"=w2422:string, "Total Header Lenght Out"=w2408:i32)  [unwired: 1 in]
        n1148 = call "Write File+ [String].vi"("String"=w2422, "error in (no error)"=w2438, "refnum"=w2439) -> ("error out"=w2428:errorcluster, "dup refnum"=w2416:refnum<file>)  [unwired: 2 in, 2 out]
        n1149 = Unbundle By Name(w2428) -> ("status"=w2431:bool, "code"=w2432:i32)
        n1150 = Equal?(x=w2432, y=w2426) -> (x = y?=w2429:bool)
        n1151 = case shown="True" w2431 {
          tunnel: [w2501 w2511] -> w2421
          tunnel: [w2500 w2512] -> w2430
          tunnel: w2429 -> [_ w2513]
          tunnel: w2428 -> [w2499 w2510]
          tunnel: [w2499 w2509] -> w2427
          tunnel: w2408 -> [w2498 w2508]
          tunnel: [w2498 w2507] -> w2407
          tunnel: w2416 -> [w2495 w2506]
          tunnel: [w2495 w2505] -> w2382
          tunnel: w2406 -> [w2489 _]
          tunnel: w2401 -> [w2492 _]
          tunnel: w2396 -> [w2493 _]
          tunnel: w2426 -> [_ w2504]
          tunnel: [T5."Enabled" ("Disabled") T5."Disabled and Grayed Out" ("Disabled")] -> w2420
          tunnel: w2414 -> [w2497 w2503]
          tunnel: [w2496 w2503] -> w2415
          tunnel: w2403 -> [w2494 _]
          tunnel: w2378 -> [w2483 _]
          tunnel: w2377 -> [w2482 _]
          tunnel: w2376 -> [w2481 _]
          frame False {
            w2501 = TRUE  # Busy Saving
            w2500 = 4  # Go to State 4: Display with Save
            n1152 = Number To Boolean Array(number=w2483) -> (Boolean array=w2488:bool[])
            n1153 = Index Array(array=w2488) -> (element #1=→"Box1":bool, element #2=→"Box2":bool, element #3=→"Box3":bool, element #4=→"Box4":bool)  [unwired: 4 in]
            n1154 = Refnum to Path(1:w2495) -> (0:w2490:path)
            n1155 = Bundle By Name(cluster=w2497, "Save Path"=w2490, "Save Subset"=w2494, "Add Touchproofs"=w2492, "Add Sensors"=w2493, "Add Jazz"=w2481, "Add Anas"=w2482, "Save Box"=w2483) -> (w2496:T7)
            n1156 = Path To String(path=w2490) -> (string=→"Filepath":string)
            "with  8 EX" <- w2492
            "with Sens" <- w2493
            "with AIB" <- w2482
            "Save Subset" <- w2489
            "with Jazz" <- w2481
          }
          frame True {
            n1157 = case shown="True" w2513 {
              tunnel: [w2518 w2530] -> w2512
              tunnel: [w2517 w2521] -> w2511
              tunnel: w2510 -> [w2516 w2527]
              tunnel: [w2516 w2528] -> w2509
              tunnel: w2508 -> [w2515 _]
              tunnel: [w2515 0 ("Total Header Lenght Out")] -> w2507
              tunnel: w2506 -> [w2514 w2523]
              tunnel: [w2514 w2519] -> w2505
              tunnel: w2504 -> [_ w2526]
              frame False {
                w2517 = TRUE  # Busy Saving
                w2518 = 5  # Go to State 5: Stop
              }
              frame True {
                w2519 = refnum<file> refnum  # Dummy Refnum
                w2520 = FALSE  # Start Saving
                w2521 = FALSE  # Busy Saving
                n1158 = Close File(refnum=w2523, error in=w2527) -> (error out=w2529:errorcluster)  [unwired: 1 out]
                n1159 = Unbundle By Name(w2529) -> ("code"=w2525:i32)
                n1160 = Equal?(x=w2526, y=w2525) -> (x = y?=w2524:bool)
                n1161 = case shown="True" w2524 {
                  tunnel: [w2532 w2534] -> w2530
                  tunnel: w2529 -> [w2531 _]
                  tunnel: [w2531 w2533] -> w2528
                  frame False {
                    w2532 = 5  # Go to State 5: Stop
                  }
                  frame True {
                    w2533 = errorcluster {"status"=FALSE, "code"=0, "source"=""}  # no error
                    w2534 = 4  # Go to State 4: Display  without Save
                  }
                }
                n1162 = local write "Start Saving"(w2520) -> ()
              }
            }
          }
        }
        n1163 = property on="Pause Saving" class="Bool (strict)"("Disabled"=w2420) -> ()  [unwired: 2 in, 2 out]
        n1164 = To Quad Integer(1:w2407) -> (0:w2384:i64)
        n1165 = local write "Pause Saving"(w2421) -> ()
      }
      frame 4 {
        w2536 = bool[] [FALSE, FALSE, FALSE, FALSE, FALSE, FALSE, FALSE, FALSE, FALSE, FALSE, FALSE, FALSE, FALSE, FALSE, FALSE]  # 15 Triggers Out
        w2623 = 0.3 ("y")
        w2642 = 1.014  # Screen Ratio
        w2681 = i32[] [] ("Initially Empty Save Array")
        w2550 = 512  # GSR/Jazz sample rate
        w2556 = FALSE  # JazzLoBatChange
        w2569 = TRUE  # Initially Filter Reset
        w2573 = FALSE  # Not Start with Save
        w2574 = FALSE  # Initialy Not Start Saving
        w2579 = 0  # Box
        w2583 = 0 ("f")
        w2606 = 3  # 3 Bytes per Sample
        w2620 = 16  # Nr of Displayed Triggers
        w2630 = FALSE
        w2663 = i16 24  # Y2
        w2661 = i16 22  # Y1
        w2664 = i16 45  # Y3
        w2666 = i16 0
        w2561 = i16 0  # Sync Errors
        w2644 = 44  # Clear Block
        w2656 = FALSE  # Initialy Not Last Call
        w2659 = 0 ("dimension size")
        w2665 = u32 13421823  # Color
        w2668 = TRUE ("fill?(F)")
        w2685 = FALSE  # LoBatChange
        w2690 = FALSE  # Second Half
        w2555 = TRUE  # Initially Filter Reset
        w2694 = i8 2  # Intiallly Screen Reset
        w2639 = 0  # Index
        w2692 = u8 0  # U8
        w2578 = i64 0  # Integer 64
        w2699 = FALSE  # Stop Running
        w2705 = 2  # Go to State 2:  Start Saving
        w2560 = FALSE  # Recent Sync Error
        w2628 = 0
        w2703 = 5  # Go to State 5: Close
        # "JazzOn"
        # "Sart with Save"
        # "Ringbuffer"
        # "Screen Duration"
        # "Config Changed"
        # "Busy Saving"
        # "Save Buffer"
        # "Busy Saving"
        # "Samples per Record"
        # "Label Cluster"
        # "Save Blocksize in Bytes"
        # "Busy Saving"
        n1166 = Unbundle By Name(w2618) -> ("Jazz Channels"=w2546:i32, "GSR16Hz"=w2553:bool, "ADC Rate"=w2551:i32, "ADC Channels"=w2558:i32, "Screen Ratio"=w2547:i32, "Decimate Ratio"=w2567:i32)
        n1167 = To Quad Integer(1:w2641) -> (0:w2577:i64)
        n1168 = To Double Precision Float(number=w2547) -> (double precision float=w2643:dbl)
        n1169 = Select(t=8 ("length"), s="TCPaddTP", f=w2583) -> (s? t:f=w2595:i32)
        n1170 = To Double Precision Float(number=w2641) -> (double precision float=w2647:dbl)
        n1171 = case shown="0, Default" "TCPsubset" {
          tunnel: [256 ("length") 160 ("length") 128 ("length") 64 ("length") 32 ("length") 16 ("length") 8 ("length") 0 ("length")] -> w2596
          frame 0, Default {
          }
          frame 1 {
          }
          frame 2 {
          }
          frame 3 {
          }
          frame 4 {
          }
          frame 5 {
          }
          frame 6 {
          }
          frame 7 {
          }
        }
        n1172 = Select(t=7, s="TCPaddSens", f=w2583) -> (s? t:f=w2594:i32)
        n1173 = Compound Arithmetic op=MULTIPLY(w2644, w2641, w2547) -> (w2646:i32)
        n1174 = Select(t=9, s="TCPaddJazz", f=w2583) -> (s? t:f=w2593:i32)
        n1175 = Not Equal To 0?(x=w2546) -> (x != 0?=w2542:bool)
        n1176 = property on="Charts/Graphs" class="TabCtl (strict)"() -> ("Pages"=w2589:refnum<vi>[])  [unwired: 2 in, 2 out]
        n1177 = Not(x=w2553) -> (.not. x?=w2548:bool)
        n1178 = To Double Precision Float(number=w2644) -> (double precision float=w2674:dbl)
        n1179 = Select(t=32, s="TCPaddAnas", f=w2583) -> (s? t:f=w2592:i32)
        n1180 = Divide(x=w2674, y=w2642) -> (x/y=w2673:dbl)
        n1181 = Select(t=1, s="TCPaddTrig", f=w2583) -> (s? t:f=w2581:i32)
        n1182 = Multiply(x=w2641, y=w2547) -> (x*y=w2619:i32)
        n1183 = Or(x=w2542, y=w2548) -> (x .or. y?=w2552:bool)
        n1184 = Quotient & Remainder(x=w2551, y=w2550) -> (floor(x/y)=w2549:i32)  [unwired: 1 out]
        n1185 = for {
          tunnel: w2589 -> [w2719] mode=indexing
          shift-right: [w2713] -> w2585
          shift-left: i32[] [] ("Disabled Items []") -> [w2715]
          i -> [w2714]
          n1186 = property class="Page"(reference=w2719) -> ("Page Enabled State"=w2718:T4)  [unwired: 1 in, 2 out]
          n1187 = Equal?(x=T4."Page Enabled" ("Page Enabled State"), y=w2718) -> (x = y?=w2716:bool)
          n1188 = case shown="False" w2716 {
            tunnel: w2715 -> [w2722 w2723]
            tunnel: w2714 -> [w2720 _]
            tunnel: [w2721 w2723] -> w2713
            frame False {
              n1189 = Build Array (concatenate)(w2722, w2720) -> (w2721:i32[])
            }
            frame True {
            }
          }
        }
        n1190 = Compound Arithmetic op=MULTIPLY(w2642, w2647, w2643) -> (w2645:dbl)
        n1191 = To Word Integer(number=w2673) -> (16bit integer=w2662:i16)
        n1192 = Select(t=w2549, s=w2552, f=w2547) -> (s? t:f=w2554:i32)
        n1193 = Quotient & Remainder(x=w2619, y=w2567) -> (floor(x/y)=w2580:i32)  [unwired: 1 out]
        n1194 = call "Act_Open.vi"("Buffer Size in Byte"=w2543, "JazzOn"=w2542) -> ("Handle Out"=w2539:i64, "Buffer Size in Words"=w2540:i64, "RingBuffer"=w2541:i32[])
        n1195 = Compound Arithmetic op=ADD(w2596, w2595, w2594, w2593, w2592, w2581) -> (w2597:i32)
        "Channels sent by TCP" <- w2597
        n1196 = Bundle("length"=w2596, "f"=w2595, "f"=w2594, "f"=w2593, "f"=w2592, "f"=w2581) -> (w2591:T24)  [unwired: 1 out]
        n1197 = Multiply(x=w2558, y=w2551) -> (x*y=w2566:i32)
        n1198 = Multiply(x=w2558, y=w2619) -> (x*y=w2609:i32)
        n1199 = Multiply(x=w2558, y=w2554) -> (x*y=w2608:i32)
        n1200 = Multiply(x=w2576, y=2) -> (x*y=w2691:i32)
        n1201 = Bundle(w2630, w2630, w2630, w2630, w2630, w2630, w2630, w2630) -> (w2629:T25)  [unwired: 1 out]
        n1202 = Bundle(w2666, w2666, w2662, "Y1"=w2661) -> (w2675:cluster{i16, i16, i16, "Y1":i16})  [unwired: 1 out]
        n1203 = Bundle By Name(cluster=T11 {"Start Averaging"=FALSE, "Busy Averaging"=FALSE, "Sweep Lenght in Samples"=0, "Valid Sweeps"=0, "Rejected Sweeps"=0, "First Graph Update"=FALSE} ("Avg Cluster In"), "Sweep Lenght in Samples"=w2637) -> (w2657:T11)
        n1204 = Multiply(x=w2606, y=w2597) -> (x*y=w2605:i32)
        n1205 = Bundle("Clear Block"=w2644, "Screen Ratio"=w2642, "Y1"=w2661, "Y2"=w2663, "Y3"=w2664, "Color"=w2665) -> (w2649:T26)  [unwired: 1 out]
        n1206 = Bundle By Name(cluster=w2649, "Clear Block"=w2646, "Screen Ratio"=w2645) -> (w2648:T26)
        n1207 = Initialize Array(w2692, w2691) -> (w2689:u8[])
        n1208 = call "Empty Picture"() -> ("empty picture"=w2672:picture)
        n1209 = Greater?(x=w2609, y=w2608) -> (0:w2610:bool)
        n1210 = property on="Channels" class="Ring (strict)"() -> ("Disabled Items []"=w2586:i32[])  [unwired: 2 in, 2 out]
        n1211 = property on="Offset" class="Ring (strict)"() -> ("Disabled Items []"=w2587:i32[])  [unwired: 2 in, 2 out]
        n1212 = call <vilib>:"Draw Rect.vi"("picture"=w2672, "rect"=w2675, "fill?(F)"=w2668, "color(black)"=w2665) -> ("new picture"=w2670:picture)  [unwired: 1 in, 4 out]
        n1213 = To Double Precision Float(number=w2620) -> (double precision float=w2621:dbl)
        n1214 = Decrement(x=w2623) -> (x-1=w2622:dbl)
        n1215 = Select(t=w2609, s=w2610, f=w2608) -> (s? t:f=w2607:i32)
        n1216 = Bundle(w2666, "Y2"=w2663, w2662, "Y3"=w2664) -> (w2667:cluster{i16, "Y2":i16, i16, "Y3":i16})  [unwired: 1 out]
        n1217 = Negate(x=w2622) -> (-x=w2625:dbl)
        n1218 = Add(x=w2621, y=w2623) -> (x+y=w2624:dbl)
        n1219 = Bundle("Sync Errors"=w2561, "Recent Sync Error"=w2560) -> (w2559:T27)  [unwired: 1 out]
        n1220 = Initialize Array(0.0 ("element"), w2659, w2659) -> (w2658:dbl[][])
        n1221 = property on="Trigger Chart" class="WFChart (strict)"("Y Scale.Range:Maximum"=w2624) -> ()  [unwired: 2 in, 2 out]
        n1222 = property on="Trigger Chart" class="WFChart (strict)"("Y Scale.Range:Minimum"=w2625) -> ()  [unwired: 2 in, 2 out]
        n1223 = To Quad Integer(1:w2566) -> (0:w2538:i64)
        n1224 = Quotient & Remainder(x=w2607, y=w2558) -> (floor(x/y)=w2617:i32)  [unwired: 1 out]
        n1225 = To Quad Integer(1:w2607) -> (0:w2537:i64)
        n1226 = call <vilib>:"Draw Rect.vi"("picture"=w2670, "rect"=w2667, "fill?(F)"=w2668, "color(black)"=w2665) -> ("new picture"=w2669:picture)  [unwired: 1 in, 4 out]
        n1227 = Select(t=1, s=w2563, f=w2628) -> (s? t:f=w2627:i32)
        n1228 = call <vilib>:"Intialize Keyboard.vi"() -> ("error out"=w2635:errorcluster, "device ID"=w2636:refnum<k1>)  [unwired: 1 in, 9 out]
        n1229 = Quotient & Remainder(x=w2617, y=w2567) -> (floor(x/y)=w2590:i32)  [unwired: 1 out]
        "TCP samples/channel" <- w2590
        n1230 = Multiply(x=w2590, y=w2605) -> (x*y=w2535:i32)
        "Bytes in TCP Array" <- w2535
        n1231 = call "AVTCP-TCP Length FGV.vi"("Value in"=w2535) -> ()  [unwired: 6 in, 1 out]
        n1232 = Bundle("LoBatChange"=w2685, "JazzLoBatChange"=w2556) -> (w2632:T28)  [unwired: 1 out]
        n1233 = To Quad Integer(1:w2576) -> (0:w2575:i64)
        n1234 = Scale By Power Of 2(n=20, x=i64 1) -> (x*2^n=w2653:i64)
        n1235 = while {
          shift-left: FALSE ("LoBatWarning") -> [w2750]
          shift-right: [w2749] -> _
          stop <- w2748 stop-if-true
          n1236 = Wait (ms)(milliseconds to wait=u32 300) -> ()  [unwired: 1 out]
          n1237 = case shown="True" w2750 {
            tunnel: [w2752 w2753] -> w2749
            frame False {
              n1238 = global read "LoBatWarning.glb" "LoBatWarning"() -> (w2752:bool)
            }
            frame True {
              n1239 = call "LoBatWarning.vi"() -> ("Ready"=w2754:bool)  [unwired: 1 out]
              n1240 = Not(x=w2754) -> (.not. x?=w2753:bool)
            }
          }
          n1241 = global read "StopThreads.glb" "StopThreads"() -> (w2748:bool)
        }
        n1242 = while {
          shift-left: FALSE ("LoBatWarning") -> [w2708]
          shift-right: [w2707] -> _
          stop <- w2706 stop-if-true
          n1243 = Wait (ms)(milliseconds to wait=u32 300) -> ()  [unwired: 1 out]
          n1244 = case shown="True" w2708 {
            tunnel: [w2710 w2711] -> w2707
            frame False {
              n1245 = global read "JazzLoBatWarning.glb" "JazzLoBatWarning"() -> (w2710:bool)
            }
            frame True {
              n1246 = call "JazzLoBatWarning.vi"() -> ("Ready"=w2712:bool)  [unwired: 1 out]
              n1247 = Not(x=w2712) -> (.not. x?=w2711:bool)
            }
          }
          n1248 = global read "StopThreads.glb" "StopThreads"() -> (w2706:bool)
        }
        n1249 = while {
          tunnel: "LocalPort" -> [w2730]
          stop <- w2728 stop-if-true
          n1250 = global read "TCPidentification.glb" "TCP cluster"() -> (w2733:T9)
          n1251 = Wait (ms)(milliseconds to wait=u32 100) -> ()  [unwired: 1 out]
          n1252 = Unbundle By Name(w2733) -> ("remote port"=w2732:u16)
          n1253 = Equal To 0?(x=w2732) -> (x = 0?=w2729:bool)
          "TCP Listening" <- w2729
          n1254 = case shown="True" w2729 {
            tunnel: w2730 -> [_ w2734]
            frame False {
            }
            frame True {
              w2735 = 1000  # timeout ms
              n1255 = call <vilib>:"TCP Listen.vi"("timeout ms (wait forever: -1)"=w2735, "port"=w2734) -> ("remote port"=w2736:u16, "remote address"=w2738:string, "connection ID"=w2739:refnum<k5>)  [unwired: 2 in, 5 out]
              n1256 = Bundle("connection ID"=w2739, "remote address"=w2738, "remote port"=w2736) -> (w2737:T9)  [unwired: 1 out]
              n1257 = global write "TCPidentification.glb" "TCP cluster"(w2737) -> ()
            }
          }
          n1258 = global read "StopThreads.glb" "StopThreads"() -> (w2728:bool)
        }
        n1259 = Unbundle By Name(w2683) -> ("Spec Labels"=w2682:string[])
        n1260 = Scale By Power Of 2(n=i16 20, x=1.0) -> (x*2^n=w2650:dbl)
        n1261 = while {
          shift-left: w2555 -> [w2986]
          shift-right: [w2985] -> _
          shift-left: w2632 -> [w2989]
          shift-right: [w2988] -> _
          shift-left: w2696 -> [w2954]
          shift-right: [w2995] -> w2695
          shift-left: w2559 -> [w3001]
          shift-right: [w3000] -> _
          shift-left: w2681 -> [w3004]
          shift-right: [w3005] -> _
          tunnel: w2682 -> [w3006]
          tunnel: w2618 -> [w2869]
          tunnel: w2576 -> [w2812]
          shift-left: w2689 -> [w2977]
          shift-right: [w3007] -> _
          shift-left: w2694 -> [w2923]
          shift-right: [w2991] -> _
          tunnel: w2563 -> [w2755]
          shift-left: w2700 -> [w2999]
          shift-right: [w3008] -> w2698
          shift-left: w2701 -> [w3009]
          shift-right: [w3010] -> w2614
          shift-left: w2697 -> [w2953]
          shift-right: [w2996] -> w2702
          tunnel: w2631 -> [w2984]
          tunnel: w2538 -> [w2994]
          shift-left: w2538 -> [w2910]
          shift-right: [w2890] -> _
          shift-left: w2628 -> [w2894]
          shift-right: [w2900] -> _
          shift-left: w2578 -> [w3002]
          shift-right: [w3014] -> _
          shift-left: w2578 -> [w3003]
          shift-right: [w2899] -> _
          tunnel: w2540 -> [w2893]
          tunnel: w2541 -> [w2891]
          shift-right: [w2983] -> _
          shift-left: w2555 -> [w2982]
          shift-right: [w2980] -> w2687
          shift-left: w2688 -> [w2981]
          tunnel: w2637 -> [w2930]
          shift-right: [w2979] -> _
          shift-left: w2639 -> [w2976]
          shift-right: [w2978] -> _
          shift-left: w2690 -> [w2834]
          tunnel: [w2761] -> w2686
          shift-right: [w2974] -> _
          shift-left: w2681 -> [w2975]
          shift-right: [w2971] -> _
          shift-left: w2555 -> [w2972]
          shift-right: [w2969] -> w2679
          shift-left: w2680 -> [w2970]
          tunnel: w2538 -> [w2905]
          tunnel: w2537 -> [w2904]
          tunnel: w2563 -> [w2816]
          shift-right: [w2957] -> w2676
          shift-left: w2677 -> [w2958]
          shift-right: [w2955] -> _
          shift-left: w2555 -> [w2956]
          shift-right: [w2948] -> _
          shift-left: w2669 -> [w2950]
          shift-right: [w2947] -> _
          shift-left: w2669 -> [w2949]
          shift-right: [w2946] -> _
          shift-left: FALSE ("fill?(F)") -> [w2943]
          tunnel: w2648 -> [w2940]
          shift-right: [w2933] -> _
          shift-left: w2658 -> [w2928]
          shift-right: [w2932] -> _
          shift-left: w2658 -> [w2929]
          shift-right: [w2931] -> _
          shift-left: w2657 -> [w2922]
          shift-right: [w2926] -> _
          shift-left: w2656 -> [w2775]
          tunnel: w2653 -> [w2909]
          tunnel: w2650 -> [w2908]
          tunnel: w2577 -> [w2906]
          tunnel: w2638 -> [w2875]
          tunnel: [w2903] -> w2640
          tunnel: w2636 -> [w2889]
          tunnel: w2635 -> [w2888]
          tunnel: [w2885] -> w2633
          tunnel: [w2884] -> w2634
          tunnel: w2586 -> [w2881]
          tunnel: w2587 -> [w2874]
          shift-right: [w2844] -> _
          shift-left: w2629 -> [w2845]
          shift-right: [w2843] -> _
          shift-left: w2628 -> [w2842]
          shift-right: [w2840] -> _
          shift-left: w2627 -> [w2841]
          tunnel: w2620 -> [w2832]
          tunnel: w2605 -> [w2831]
          tunnel: w2590 -> [w2830]
          tunnel: [w2824] -> w2612
          tunnel: [w2826] -> w2611
          tunnel: w2591 -> [w2825]
          tunnel: w2585 -> [w2820]
          tunnel: w2580 -> [w2819]
          shift-right: [w2817] -> _
          shift-left: w2579 -> [w2818]
          tunnel: w2575 -> [w2811]
          shift-right: [w2815] -> w2564
          shift-left: w2574 -> [w2807]
          tunnel: w2572 -> [w2806]
          shift-right: [w2802] -> _
          shift-left: T2."Monopolar Display" ("Charts/Graphs") -> [w2803]
          shift-right: [w2798] -> w2568
          shift-left: w2570 -> [w2799]
          shift-right: [w2796] -> _
          shift-left: w2569 -> [w2797]
          shift-right: [w2769] -> _
          shift-left: w2536 -> [w2768]
          tunnel: [w2770] -> w2544
          tunnel: w2539 -> [w2766]
          i -> [w2897]
          stop <- w2775 stop-if-true
          w2767 = T2."Event Related Average" ("Charts/Graphs")
          w2862 = T29 [] items=["0", "1", "2", "3", "4", "5", "6", "7", "8", "9", "A", "B", "C", "D", "E", "F", "G", "H", "I", "J", "K", "L", "M", "N", "O", "P", "Q", "R", "S", "T", "U", "V", "W", "X", "Y", "Z", "F1", "F2", "F3", "F4", "F5", "F6", "F7", "F8", "F9", "F10", "F11", "F12", "F13", "F14", "F15", "ADD", "BACK", "BACKSLASH", "CAPITAL", "COMMA", "DECIMAL", "DELETE", "DIVIDE", "DOWN", "END", "EQUALS", "ESCAPE", "GRAVE (`)", "HOME", "INSERT", "LBRACKET", "LCONTROL", "LEFT", "L ALT", "LSHIFT", "LWIN", "MINUS", "MULTIPLY", "NEXT", "NUMLOCK", "NUMPAD_0", "NUMPAD_1", "NUMPAD_2", "NUMPAD_3", "NUMPAD_4", "NUMPAD_5", "NUMPAD_6", "NUMPAD_7", "NUMPAD_8", "NUMPAD_9", "PAUSE", "PERIOD", "PRIOR (PG UP)", "RBRACKET", "RCONTROL", "RETURN", "RIGHT", "R ALT", "RSHIFT", "RWIN", "SCROLL", "SEMICOLON", "SLASH", "SPACE", "SUBTRACT", "TAB", "UP", "ENTER (num pad)", "' (quote)"] ("f")
          w2927 = i8 4  # Avg
          w2997 = i8 3  # EOF
          w3011 = i8 2  # Save
          w3012 = i8 1  # Display
          w3013 = i8 0  # Wait
          (unwired) 32
          # "Speed/Save Cluster"
          # "Average Total"
          # "Noise Total"
          # "Total ADC Sample/s"
          # "Jazz Channel Selection"
          # "Jazz Filter Reset"
          # "Jazz Channel Selection"
          # "Jazz Filter Reset"
          # "Box"
          # "Box"
          # "Save Blocksize in Bytes"
          # "File Limit in Byte"
          # "Time Limit"
          # "Number of Files"
          # "Number of Files"
          # "Total Saved in Sec"
          # "Total Saved in Sec"
          # "Markers"
          # "Driver Handle"
          # "Handle"
          # "System Cluster"
          # "Extra Blocksize Check"
          # "Buffer pointer in Byte"
          # "in Mbyte"
